vi "TestInitializeBasicPolicy_PublishOK.vi"(8 "error in (no error)":errorcluster, 11 "TestCase in":refnum<class "TestSubscriptionPolicy.lvclass">) -> (0 "error out":errorcluster, 3 "TestCase out":refnum<class "TestSubscriptionPolicy.lvclass">)   [LabVIEW 2015, in "SubscriptionPolicy.lvlib" / "TestSubscriptionPolicy.lvclass"]
uses:
  TestSubscriptionPolicy.lvclass
  BasicSubscription/BasicSubscription.lvclass/BasicSubscription.ctl
  BasicSubscription/BasicSubscription.lvclass
  IMediator/ISubscriptionPolicy/ISubscriptionPolicy.lvclass
  Transport/QueueTransport/QueueTransport.lvclass
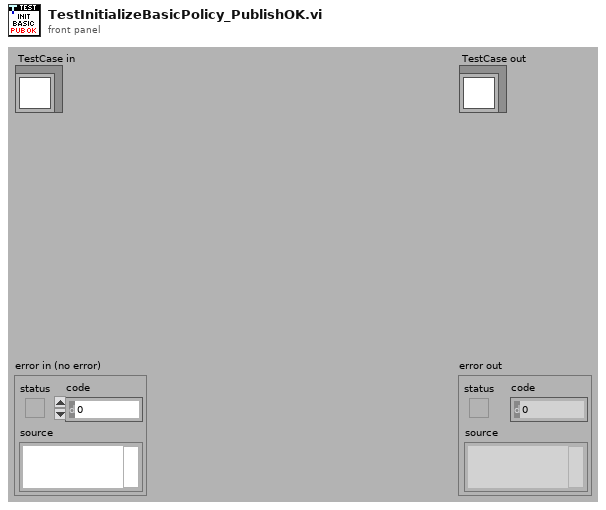
[diagram p1: front panel]
types:
  T1 = typedef "IMediator.lvlib/ISubscriptionPolicy.lvclass/ISubscriptionPolicy Reference.ctl" = refnum<data-value>
  T2 = cluster{"Data":variant, "Publication Time":timestamp}
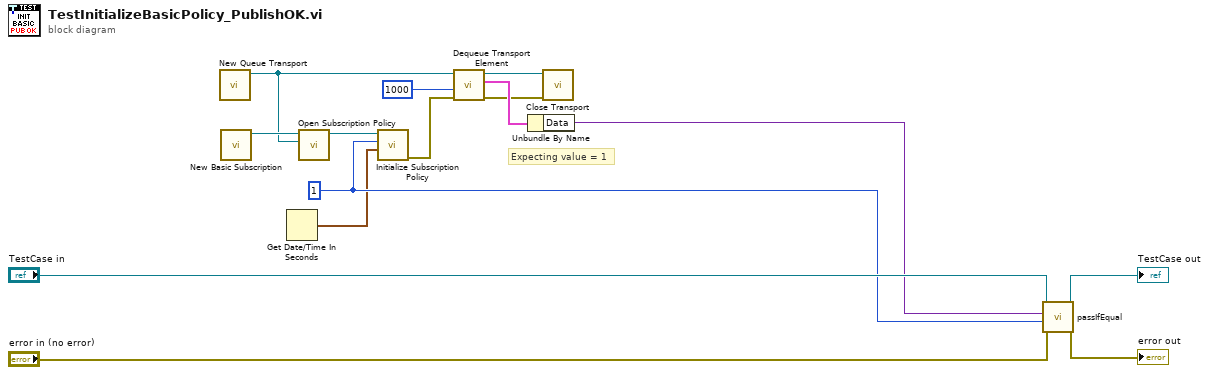
[diagram p0: block diagram]
diagram:
  w6 = 1
  # "Expecting value = 1"
  n1 = call "New Queue Transport.vi"() -> ("QueueTransport Out"=w1:refnum<class "QueueTransport.lvclass">)  [unwired: 10 in, 1 out]
  n2 = call "New Basic Subscription.vi"() -> ("BasicSubscription Out"=w2:refnum<class "BasicSubscription.lvclass">)  [unwired: 11 in]
  n3 = Get Date/Time In Seconds() -> (seconds since 1Jan1904=w5:timestamp)
  n4 = call "Open Subscription Policy.vi"("Transport"=w1, "SubscriptionPolicy"=w2) -> ("Subscription Policy"=w11:T1)  [unwired: 8 in, 1 out]
  n5 = call "Initialize Subscription Policy.vi"("Last Publish Time"=w5, "Last Topic Value"=w6, "Subscription Policy"=w11) -> ("Error Out (Do Not Subscribe?)"=w10:errorcluster)  [unwired: 8 in]
  n6 = call "Dequeue Transport Element.vi"("error in (no error)"=w10, "Timeout In ms (-1)"=1000, "QueueTransport in"=w1) -> ("error out"=w3:errorcluster, "Element"=w8:T2, "QueueTransport out"=w4:refnum<class "QueueTransport.lvclass">)  [unwired: 5 in, 1 out]
  n7 = Unbundle By Name(w8) -> ("Data"=w7:variant)
  n8 = call-dynamic "Close Transport.vi"("error in (no error)"=w3, "QueueTransport in"=w4) -> ()  [unwired: 9 in, 1 out]
  n9 = call-dynamic "passIfEqual.vi"("error in (no error)"="error in (no error)", "y"=w6, "x"=w7, "TestCase in"="TestCase in") -> ("error out"=→"error out":errorcluster, "TestCase out"=→"TestCase out":refnum<class "TestSubscriptionPolicy.lvclass">)  [unwired: 6 in]
